vi "Share Stop Signal (sub-vi).vi"(0 "set stop (F)":bool, 1 "channel":T1) -> (2 "stop":bool)   [LabVIEW 2021]
doc: "Use this VI to stop multiple parallel loops when there is not an existing way of communicating between those loops that can carry the stop signal (it is generally better to carry the stop signal in the same medium as all the other data to avoid race conditions and deadlocks). \n\nThis VI will return <b>stop</b> as TRUE if <b>set stop</b> is TRUE or if the <b>channel</b> has been set to TRUE by another call to this VI."
uses:
  <extravilib>/ChannelInstances/Tag-bool/))Channel.ctl
  <extravilib>/ChannelInstances/Tag-bool/Read With Abort.vi
  <extravilib>/ChannelInstances/Tag-bool/Write With Abort.vi
  <extravilib>/ChannelInstances/Tag-bool/EndpointRead.vi
  <extravilib>/ChannelInstances/Tag-bool/Endpoint.vi
  <extravilib>/ChannelInstances/Tag-bool.lvlib
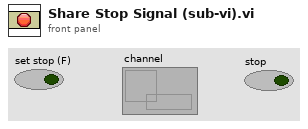
[diagram p1: front panel]
types:
  T1 = typedef "Tag-bool.lvlib/))Channel.ctl" = refnum<queue>
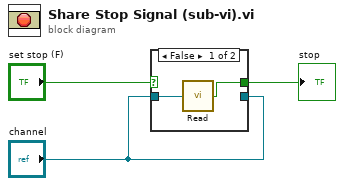
[diagram p0: block diagram]
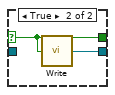
[diagram p2: hidden frame]
diagram:
  n1 = case shown="False" "set stop (F)" {
    selector: "set stop (F)" -> [_ w6]
    tunnel: [w5 w6] -> w3
    tunnel: "channel" -> [_ w7]
    tunnel: "channel" -> [w4 _]
    frame False {
      n2 = call <extravilib>:"Read.vi"("channel"=w4) -> ("element"=w5:bool)  [unwired: 1 in, 1 out]
    }
    frame True {
      n3 = call <extravilib>:"Write.vi"("element"=w6) -> ("channel"=w7:T1)  [unwired: 1 out]
    }
  }
  "stop" <- w3
